vi "DecodeQDC.vi"(11 "Buff":u32[](array[numeric])) -> (2 "Error Read Value":u32 format="%.0x", 3 "Array":T1(array[cluster]))   [LabVIEW 2014]
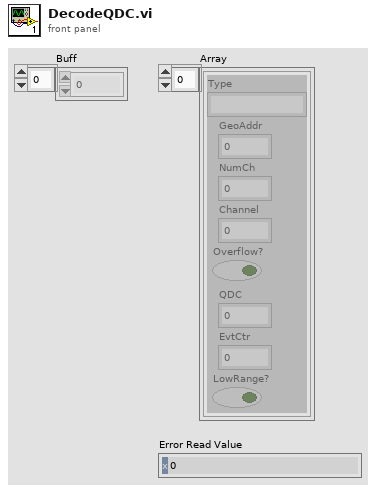
[diagram p1: front panel]
types:
  T1 = cluster{"Type":string, "GeoAddr":u8, "NumCh":u8, "Channel":u8, "Overflow?":bool, "QDC":u16, "EvtCtr":u32, "LowRange?":bool}[]
  T2 = cluster{"Type":string, "GeoAddr":u8, "NumCh":u8, "Channel":u8, "Overflow?":bool, "QDC":u16, "EvtCtr":u32, "LowRange?":bool}
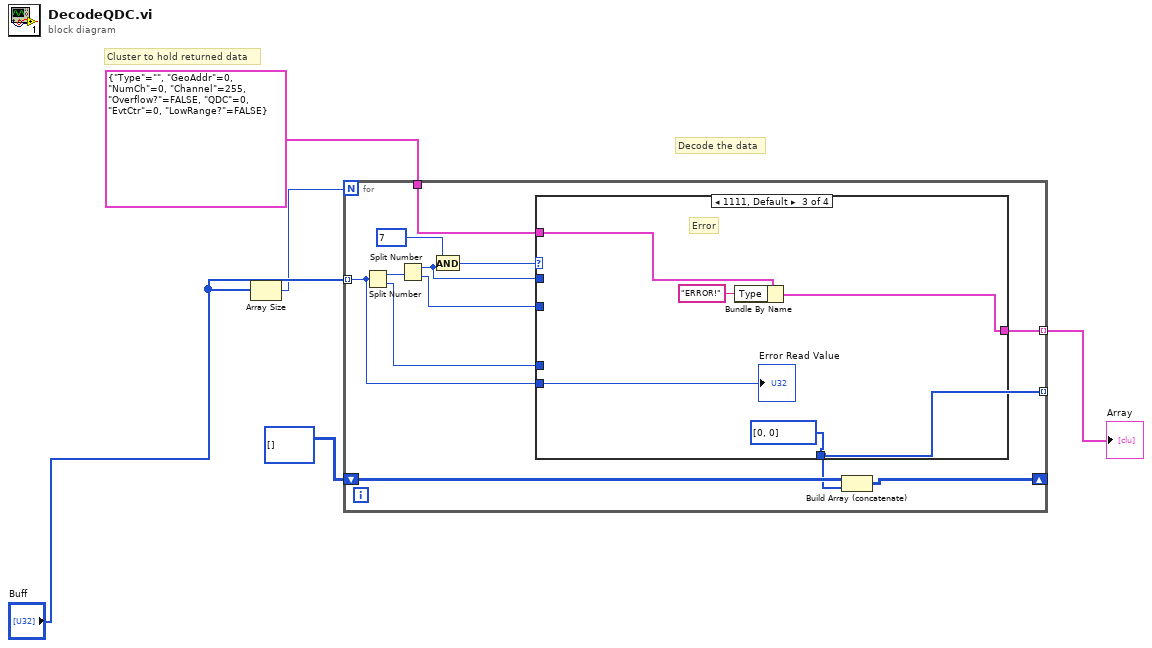
[diagram p0: block diagram]
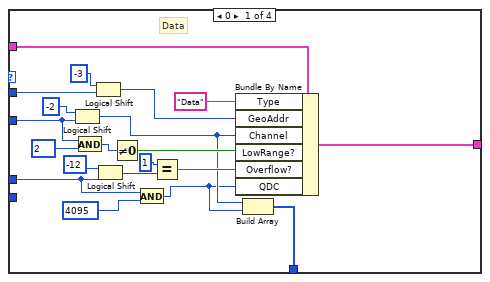
[diagram p2: hidden frame]
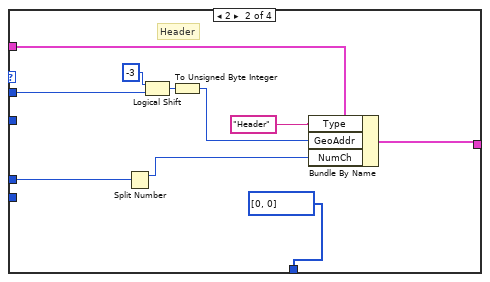
[diagram p3: hidden frame]
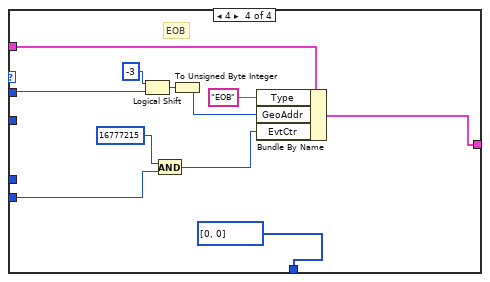
[diagram p4: hidden frame]
diagram:
  # "Decode the data"
  # "Cluster to hold returned data"
  n1 = Array Size(array="Buff") -> (size(s)=w1:i32)
  n2 = for {
    N: w1 -> [_]
    tunnel: "Buff" -> [w11] mode=indexing
    tunnel: T2 {"Type"="", "GeoAddr"=0, "NumCh"=0, "Channel"=255, "Overflow?"=FALSE, "QDC"=0, "EvtCtr"=0, "LowRange?"=FALSE} -> [w14]
    tunnel: [w9] -> w3 mode=indexing
    tunnel: [w7] -> _ mode=indexing
    shift-right: [w6] -> _
    shift-left: u32[][] [] -> [w8]
    n3 = Split Number(x=w11) -> (hi(x)=w17:u16, lo(x)=w12:u16)
    n4 = Split Number(x=w17) -> (hi(x)=w13:u8, lo(x)=w10:u8)
    n5 = And(x=u8 7, y=w13) -> (x .and. y?=w15:u8)
    n6 = case shown="1111, Default" w15 {
      tunnel: w14 -> [w37 w43 w52 w63]
      tunnel: w13 -> [w34 w47 _ w59]
      tunnel: w12 -> [w26 w44 _ _]
      tunnel: w11 -> [_ _ w50 w57]
      tunnel: w10 -> [w32 _ _ _]
      tunnel: [w24 w39 w49 w54] -> w9
      tunnel: [w18 u32[] [0, 0] ("Buff") u32[] [0, 0] ("Buff") u32[] [0, 0] ("Buff")] -> w7
      frame 0 {
        # "Data"
        n7 = Logical Shift(y=i16 -2, x=w32) -> (x << y=w20:u8)
        n8 = And(x=w32, y=u8 2) -> (x .and. y?=w30:u8)
        n9 = Logical Shift(y=i16 -3, x=w34) -> (x << y=w28:u8)
        n10 = Logical Shift(y=i16 -12, x=w26) -> (x << y=w23:u16)
        n11 = Not Equal To 0?(x=w30) -> (x != 0?=w29:bool)
        n12 = And(x=w26, y=u16 4095) -> (x .and. y?=w19:u16)
        n13 = Equal?(x=u16 1, y=w23) -> (x = y?=w21:bool)
        n14 = Bundle By Name(cluster=w37, "Type"="Data", "GeoAddr"=w28, "Channel"=w20, "LowRange?"=w29, "Overflow?"=w21, "QDC"=w19) -> (w24:T2)
        n15 = Build Array(w20, w19) -> (w18:u16[])
      }
      frame 2 {
        # "Header"
        n16 = Split Number(x=w44) -> (hi(x)=w40:u8)  [unwired: 1 out]
        n17 = Logical Shift(y=i16 -3, x=w47) -> (x << y=w45:u8)
        n18 = To Unsigned Byte Integer(number=w45) -> (unsigned 8bit integer=w41:u8)
        n19 = Bundle By Name(cluster=w43, "Type"="Header", "GeoAddr"=w41, "NumCh"=w40) -> (w39:T2)
      }
      frame 15, Default {
        # "Error"
        n20 = Bundle By Name(cluster=w52, "Type"="ERROR!") -> (w49:T2)
        "Error Read Value" <- w50
      }
      frame 4 {
        # "EOB"
        n21 = Logical Shift(y=i16 -3, x=w59) -> (x << y=w61:u8)
        n22 = And(x=u32 16777215, y=w57) -> (x .and. y?=w55:u32)
        n23 = To Unsigned Byte Integer(number=w61) -> (unsigned 8bit integer=w58:u8)
        n24 = Bundle By Name(cluster=w63, "Type"="EOB", "GeoAddr"=w58, "EvtCtr"=w55) -> (w54:T2)
      }
    }
    n25 = Build Array (concatenate)(w8, w7) -> (w6:u32[][])
  }
  "Array" <- w3
